vi "test.vi"() -> ()   [LabVIEW 2016]
uses:
  Typedefs/GratingType.ctl
  Typedefs/AckType.ctl
  Typedefs/slit.ctl
  Typedefs/SlitType.ctl
  Typedefs/slitWidth.ctl
  Typedefs/wavelength.ctl
  MonoClient/MonoClientCommunicator.lvclass
  ts_labview_tcp/TCPClient/TCPClient.lvclass
  home/andres/ts_monochromator/ss_monochromator/ts_labview_tcp/TCPCommunicator/TCPCommunicator.lvclass
  ts_labview_tcp/TCPSettings/TCPSettings.lvclass
  ts_labview_tcp/tcpTypedefs/TCPSettings.ctl
  ts_labview_tcp/TCPCommunicator/TCPCommunicator.lvclass/TCPCommunicator.ctl
  MonoClient/MonoClientCommunicator.lvclass/MonoClientCommunicator.ctl
  ts_labview_tcp/TCPComEvents/TCPComEvents.lvclass
  ts_labview_tcp/TCPCommunicator/TCPCommunicator.lvclass
panel:
  in  "wavelength":T1=4.0000000000000003e-07
  in  "Reset":bool
  in  "SlitType":T2
  out "slitWidth":T3
  out "Grating":T4
  out "wavelength 2":T1=4.0000000000000003e-07
  in  "slitPosition":T5
  out "Ack":T6
  out "error out":errorcluster
  in  "GratingType":T4
  in  "Get Slit Width":bool
  in  "Get Grating":bool
  in  "Get Wavelength":bool
  in  "Set Slit Width":bool
  in  "Set Grating":bool
  in  "Calibrate Wavelength":bool
  in  "Set Wavelength":bool
  in  "stop":bool
  # "Inputs"
  # "Outputs"
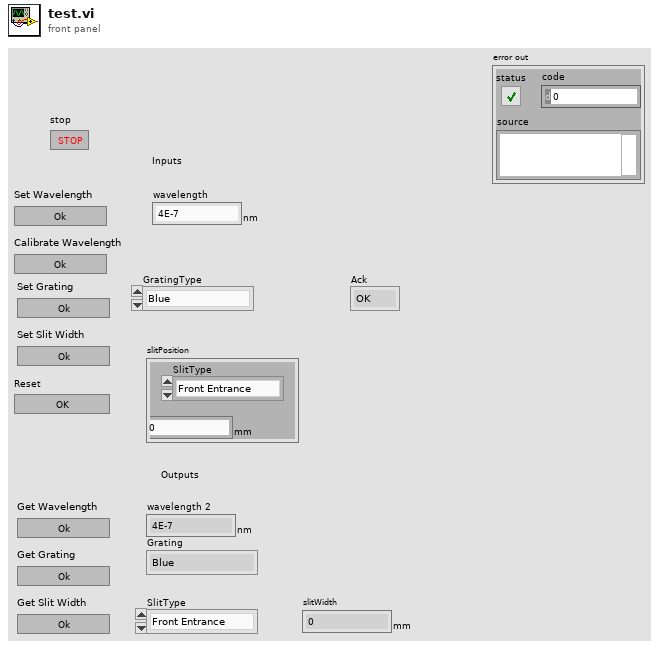
[diagram p1: front panel]
types:
  T1 = typedef "wavelength.ctl" = dbl[unit]
  T2 = typedef "SlitType.ctl" = enum16{"Front Entrance", "Side Entrance", "Front Exit", "Side Exit", "First Intermediate", "Second Intermediate"}
  T3 = typedef "slitWidth.ctl" = dbl[unit]
  T4 = typedef "GratingType.ctl" = enum16{"Blue", "Red", "Mirror"}
  T5 = typedef "slit.ctl" = cluster{"SlitType":T2, "Width":T3}
  T6 = typedef "AckType.ctl" = enum16{"OK", "OutOfRange", "Unknown", "Busy", "Rejected"}
  T7 = typedef "TCPSettings.ctl" = cluster{"IP":string, "port_low":u16, "port_up":u16, "connection_timeout ":i32, "reading_timeout":i32, "writing_timeout":i32}
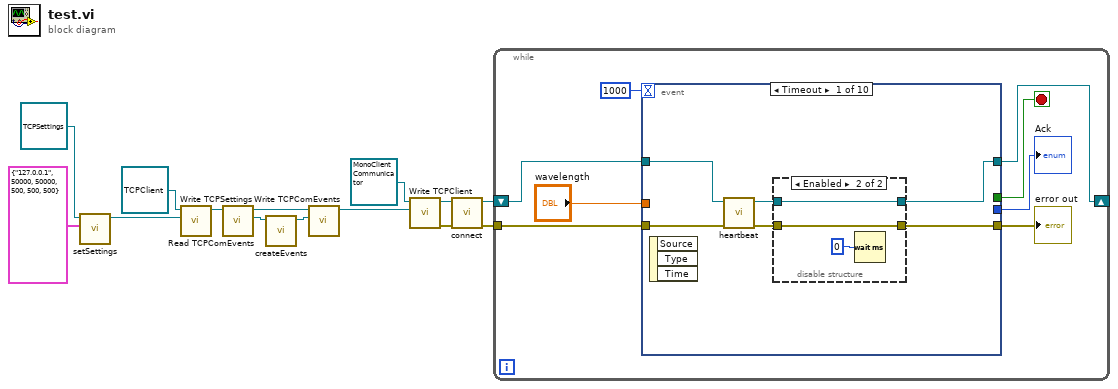
[diagram p0: block diagram]
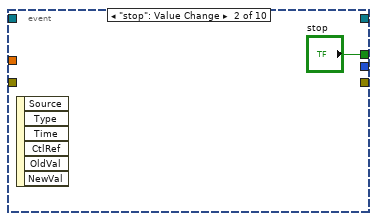
[diagram p3: hidden frame]
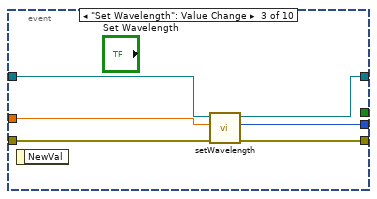
[diagram p4: hidden frame]
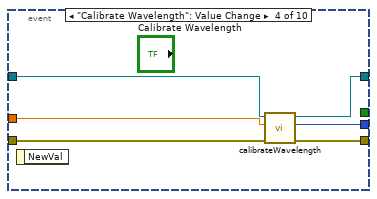
[diagram p5: hidden frame]
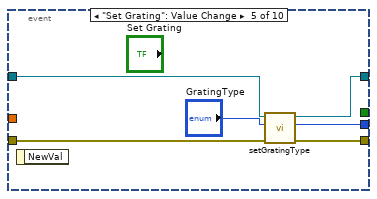
[diagram p6: hidden frame]
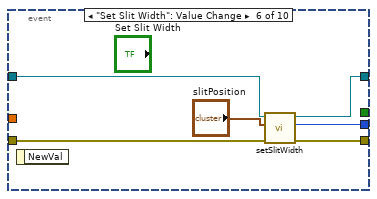
[diagram p7: hidden frame]
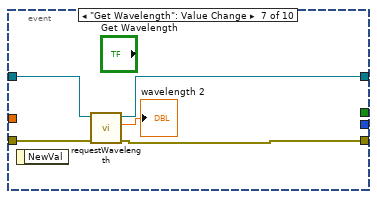
[diagram p8: hidden frame]
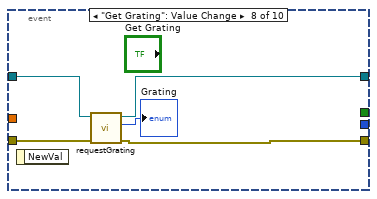
[diagram p9: hidden frame]
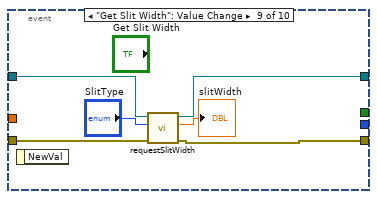
[diagram p10: hidden frame]
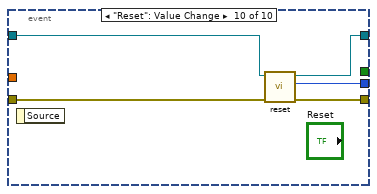
[diagram p11: hidden frame]
diagram:
  n1 = call "setSettings.vi"("Settings"=T7 {"IP"="127.0.0.1", "port_low"=50000, "port_up"=50000, "connection_timeout "=500, "reading_timeout"=500, "writing_timeout"=500}, "TCPSettings in"=refnum<class "TCPSettings.lvclass"> refnum ("TCPSettings.lvclass")) -> ("TCPSettings out"=w12:refnum<class "TCPSettings.lvclass">)  [unwired: 8 in, 1 out]
  n2 = call-dynamic "Write TCPSettings.vi"("TCPSettings.lvclass"=w12, "TCPCommunicator in"=refnum<class "TCPClient.lvclass"> refnum ("TCPClient.lvclass")) -> ("TCPCommunicator out"=w5:refnum<class "TCPClient.lvclass">)  [unwired: 8 in, 1 out]
  n3 = call "Read TCPComEvents.vi"("TCPCommunicator in"=w5) -> ("TCPComEvents.lvclass"=w4:refnum<class "TCPComEvents.lvclass">, "TCPCommunicator out"=w3:refnum<class "TCPClient.lvclass">)  [unwired: 8 in, 1 out]
  n4 = call "createEvents.vi"("TCPComEvents in"=w4) -> ("TCPComEvents out"=w2:refnum<class "TCPComEvents.lvclass">)  [unwired: 9 in, 1 out]
  n5 = call "Write TCPComEvents.vi"("TCPComEvents.lvclass"=w2, "TCPCommunicator in"=w3) -> ("TCPCommunicator out"=w1:refnum<class "TCPClient.lvclass">)  [unwired: 8 in, 1 out]
  n6 = call "Write TCPClient.vi"("TCPClient.lvclass"=w1, "MonoClient in"=refnum<class "MonoClientCommunicator.lvclass"> refnum ("MonoClientCommunicator.lvclass")) -> ("error out"=w8:errorcluster, "MonoClient out"=w10:refnum<class "MonoClientCommunicator.lvclass">)  [unwired: 8 in]
  n7 = call "connect.vi"("error in (no error)"=w8, "MonoClientCommunicator in"=w10) -> ("error out"=w7:errorcluster, "MonoClientCommunicator out"=w9:refnum<class "MonoClientCommunicator.lvclass">)  [unwired: 8 in]
  n8 = while {
    tunnel: w7 -> [w19]
    shift-right: [w18] -> _
    shift-left: w9 -> [w20]
    stop <- w21 stop-if-true
    n9 = event shown="[0] Timeout" {
      selector: _ -> [_ _ _ _ _ _ _ _ _ _]
      dyn-events: _ -> [_ _ _ _ _ _ _ _ _ _]
      timeout: 1000 -> [_ _ _ _ _ _ _ _ _ _]
      tunnel: [_ "stop" _ _ _ _ _ _ _ _] -> w21
      tunnel: w20 -> [w28 _ w40 w46 w47 w58 w63 w68 w74 w79]
      tunnel: "wavelength" -> [_ _ w36 w45 _ _ _ _ _ _]
      tunnel: w19 -> [w27 _ w37 w44 w49 w54 w60 w67 w71 w78]
      tunnel: [w25 _ w38 w43 w50 w56 w61 w66 w72 w77] -> w17
      tunnel: [w23 _ w39 w42 w52 w57 w62 w65 w73 w76] -> w18
      tunnel: [_ _ w35 w41 w51 w55 _ _ _ w75] -> w16
      event Timeout {
        n10 = event-data() -> ()  [unwired: 1 in, 3 out]
        n11 = call "heartbeat.vi"("error in (no error)"=w27, "MonoClientCommunicator in"=w28) -> ("error out"=w26:errorcluster, "MonoClientCommunicator out"=w24:refnum<class "MonoClientCommunicator.lvclass">)  [unwired: 6 in, 2 out]
        n12 = disable-structure shown="Enabled" {
          disable-tunnel: w26 -> [w29 w33]
          disable-tunnel: [w29 w33] -> w25
          disable-tunnel: [w30 w32] -> w23
          disable-tunnel: w24 -> [w30 w32]
          frame Disabled {
          }
          frame Enabled {
            n13 = Wait (ms)(milliseconds to wait=u32 0) -> ()  [unwired: 1 out]
          }
        }
      }
      event "stop": Value Change {
        n14 = event-data() -> ()  [unwired: 1 in, 6 out]
      }
      event "Set Wavelength": Value Change {
        n15 = event-data() -> ()  [unwired: 1 in, 1 out]
        n16 = call "setWavelength.vi"("error in (no error)"=w37, "wavelength"=w36, "MonoClientCommunicator in"=w40) -> ("error out"=w38:errorcluster, "ack"=w35:T6, "MonoClientCommunicator out"=w39:refnum<class "MonoClientCommunicator.lvclass">)  [unwired: 6 in]
      }
      event "Calibrate Wavelength": Value Change {
        n17 = event-data() -> ()  [unwired: 1 in, 1 out]
        n18 = call "calibrateWavelength.vi"("error in (no error)"=w44, "wavelength"=w45, "MonoClientCommunicator in"=w46) -> ("error out"=w43:errorcluster, "Ack"=w41:T6, "MonoClientCommunicator out"=w42:refnum<class "MonoClientCommunicator.lvclass">)  [unwired: 6 in]
      }
      event "Set Grating": Value Change {
        n19 = event-data() -> ()  [unwired: 1 in, 1 out]
        n20 = call "setGratingType.vi"("error in (no error)"=w49, "GratingType"="GratingType", "MonoClientCommunicator in"=w47) -> ("error out"=w50:errorcluster, "ack"=w51:T6, "MonoClientCommunicator out"=w52:refnum<class "MonoClientCommunicator.lvclass">)  [unwired: 6 in]
      }
      event "Set Slit Width": Value Change {
        n21 = event-data() -> ()  [unwired: 1 in, 1 out]
        n22 = call "setSlitWidth.vi"("error in (no error)"=w54, "position"="slitPosition", "MonoClientCommunicator in"=w58) -> ("error out"=w56:errorcluster, "ack"=w55:T6, "MonoClientCommunicator out"=w57:refnum<class "MonoClientCommunicator.lvclass">)  [unwired: 6 in]
      }
      event "Get Wavelength": Value Change {
        n23 = event-data() -> ()  [unwired: 1 in, 1 out]
        n24 = call "requestWavelength.vi"("error in (no error)"=w60, "MonoClientCommunicator in"=w63) -> ("error out"=w61:errorcluster, "wavelength"=→"wavelength 2":T1, "MonoClientCommunicator out"=w62:refnum<class "MonoClientCommunicator.lvclass">)  [unwired: 7 in]
      }
      event "Get Grating": Value Change {
        n25 = event-data() -> ()  [unwired: 1 in, 1 out]
        n26 = call "requestGrating.vi"("error in (no error)"=w67, "MonoClientCommunicator in"=w68) -> ("error out"=w66:errorcluster, "Grating"=→"Grating":T4, "MonoClientCommunicator out"=w65:refnum<class "MonoClientCommunicator.lvclass">)  [unwired: 7 in]
      }
      event "Get Slit Width": Value Change {
        n27 = event-data() -> ()  [unwired: 1 in, 1 out]
        n28 = call "requestSlitWidth.vi"("error in (no error)"=w71, "SlitType"="SlitType", "MonoClientCommunicator in"=w74) -> ("error out"=w72:errorcluster, "slitWidth"=→"slitWidth":T3, "MonoClientCommunicator out"=w73:refnum<class "MonoClientCommunicator.lvclass">)  [unwired: 6 in]
      }
      event "Reset": Value Change {
        n29 = event-data() -> ()  [unwired: 1 in, 1 out]
        n30 = call "reset.vi"("error in (no error)"=w78, "MonoClientCommunicator in"=w79) -> ("error out"=w77:errorcluster, "ack"=w75:T6, "MonoClientCommunicator out"=w76:refnum<class "MonoClientCommunicator.lvclass">)  [unwired: 7 in]
      }
    }
    "error out" <- w17
    "Ack" <- w16
  }
